vi "KlingerV2 SetZero.vi"(0 "VISA Rsrc":refnum<visa-resource-name>="SR530", 1 "Position Ref":refnum<vi>, 2 "Axe":u8(ring) items=["W", "X", "Y", "Z"], 3 "error in":errorcluster, 4 "UnitDem":u8(ring)=2 caption="Unités" items=["Pas", "mm", "ps"]) -> (5 "Statut":bool, 6 "Ind Comm":string, 7 "error out":errorcluster)   [LabVIEW 2019]
doc: "Ce Vi définit la position actuelle de l'axe spécifié comme zéro."
panel:
  out "Message D'erreur":string
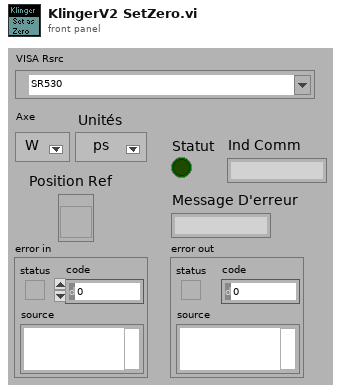
[diagram p1: front panel]
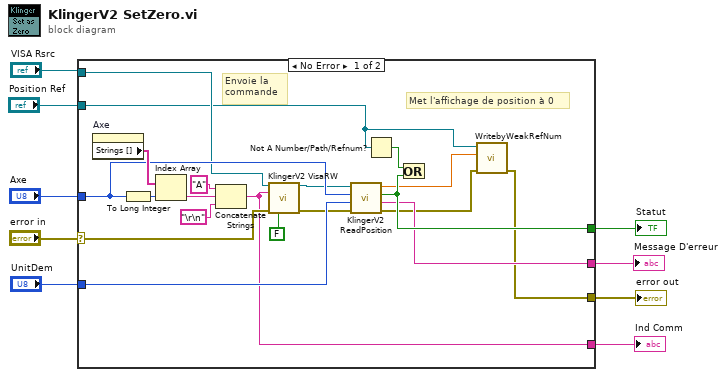
[diagram p0: block diagram]
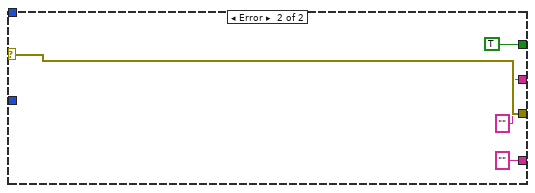
[diagram p2: hidden frame]
diagram:
  n1 = case shown="No Error" "error in" {
    selector: "error in" -> [w16 w33]
    tunnel: [w15 ""] -> w9
    tunnel: "Axe" -> [w21 _]
    tunnel: "Position Ref" -> [w13 _]
    tunnel: [w23 TRUE ("Statut")] -> w6
    tunnel: [w10 w33] -> w5
    tunnel: [w22 "" ("Message D'erreur")] -> w4
    tunnel: "VISA Rsrc" -> [w17 _]
    tunnel: "UnitDem" -> [w20 _]
    frame No Error {
      # "Envoie la \ncommande"
      # "Met l'affichage de position à 0"
      n2 = property on="Axe" class="MDér (strict)"() -> ("Strings []"=w27:string[])  [unwired: 2 in, 2 out]
      n3 = To Long Integer(number=w21) -> (32bit integer=w26:i32)
      n4 = Index Array(array=w27, index=w26) -> (element=w25:string)
      n5 = Concatenate Strings("A", w25, "\r\n") -> (w15:string)
      n6 = call <userlib>:"KlingerV2 VisaRW.vi"("VISA Rsrc"=w17, "ChaineCom"=w15, "error in (no error)"=w16, "Lecture?(T)"=FALSE) -> ("VISA Rsrc Out"=w19:refnum<visa-resource-name>, "error out"=w18:errorcluster)  [unwired: 7 in, 3 out]
      n7 = call <userlib>:"KlingerV2 ReadPosition.vi"("error in"=w18, "UnitDem"=w20, "Axe"=w21, "VISA Rsrc"=w19) -> ("error out"=w11:errorcluster, "Cont Error"=w22:string, "Statut"=w23:bool, "Position"=w12:dbl)  [unwired: 1 in, 3 out]
      n8 = Not A Number/Path/Refnum?(number/path/refnum=w13) -> (NaN/Path/Refnum?=w24:bool)
      n9 = Or(x=w24, y=w23) -> ()  [unwired: 1 out]
      n10 = call <userlib>:"WritebyWeakRefNum.vi"("error in"=w11, "Valeur"=w12, "Control Ref"=w13) -> ("error out"=w10:errorcluster)  [unwired: 8 in]
    }
    frame Error {
    }
  }
  "error out" <- w5
  "Ind Comm" <- w9
  "Message D'erreur" <- w4
  "Statut" <- w6
